vi "GetFrameCountSinceStart.vi"(0 "object in":refnum<class "Hamamatsu.lvclass">, 5 "error in (no error)":errorcluster) -> (14 "object out":refnum<class "Hamamatsu.lvclass">, 15 "FrameCountSinceStart":i32, 16 "FramesPerAquisionCycle":i32, 19 "error out":errorcluster)   [LabVIEW 2021, in "Hamamatsu.lvclass"]
uses:
  Hamamatsu.lvclass
  Hamamatsu.lvclass/Hamamatsu.ctl
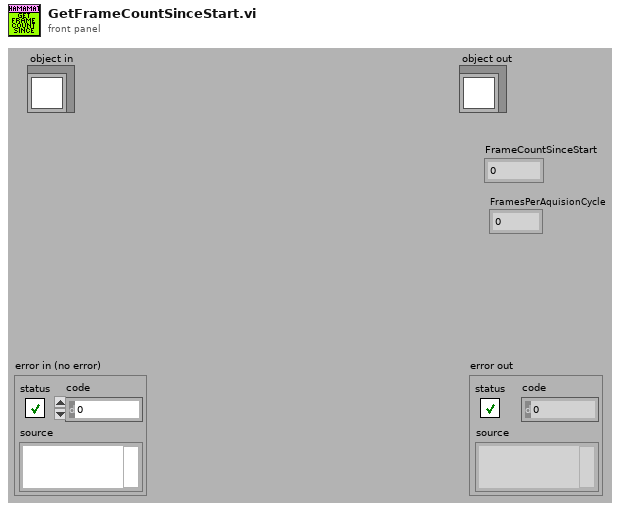
[diagram p1: front panel]
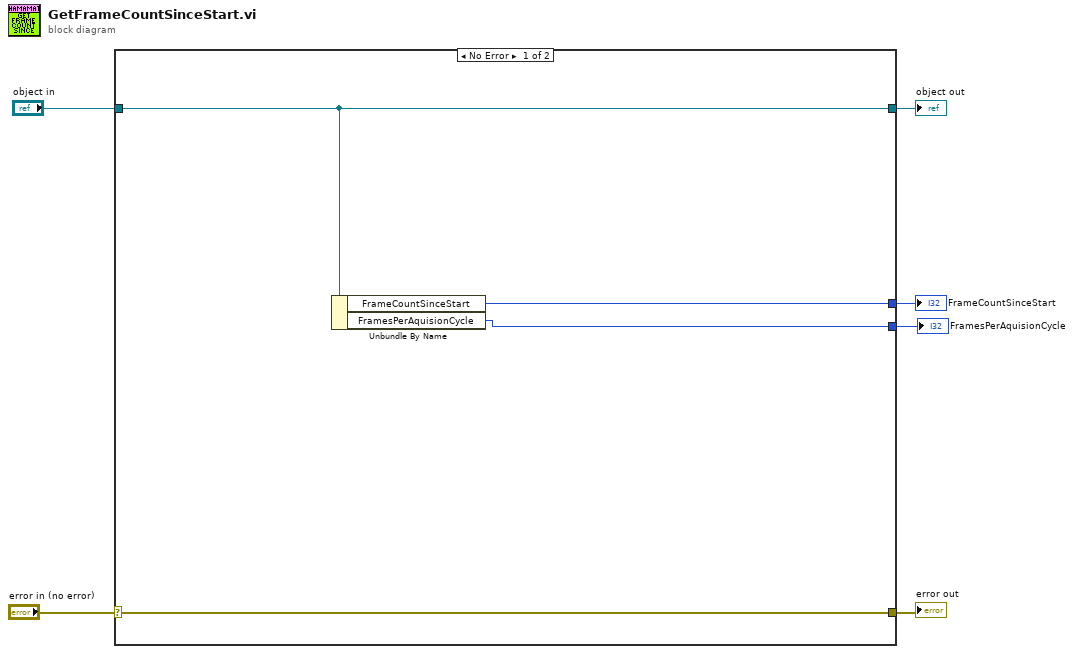
[diagram p0: block diagram]
diagram:
  n1 = case shown="No Error" "error in (no error)" {
    selector: "error in (no error)" -> [w9 w12]
    tunnel: [w9 w12] -> w5
    tunnel: [w8 w11] -> w3
    tunnel: "object in" -> [w8 w11]
    tunnel: [w10 _] -> w2
    tunnel: [w7 _] -> w1
    frame No Error {
      n2 = Unbundle By Name(w8) -> ("FrameCountSinceStart"=w10:i32, "FramesPerAquisionCycle"=w7:i32)
    }
    frame Error {
    }
  }
  "error out" <- w5
  "object out" <- w3
  "FrameCountSinceStart" <- w2
  "FramesPerAquisionCycle" <- w1
